vi "Raycaster_DrawBackground.vi"(7 "column":u32) -> ()   [LabVIEW 2020]
uses:
  <vilib>/Platform/TimedLoop/XDataNode/timing_clust.ctl
  <vilib>/Platform/TimedLoop/XDataNode/nitl_modes.ctl
  <vilib>/Platform/TimedLoop/XDataNode/wakeup.ctl
  <vilib>/rvi/Emulation/niFpgaEmulationIsFPGAContextNoSignature.vi
  <vilib>/rvi/DataTransferAndStorage/Container/Common/niFpgaContainerGetUniqueNameForEmu.vi
  <vilib>/rvi/Memory/Memory_Emulation/niFpgaMemoryEmulationCacheClearOnFirstRun.vi
  <vilib>/rvi/Memory/Memory_Emulation/nirvimemoryEmulationManagerCache_MakeExclusive.vi
  <vilib>/rvi/Memory/Memory_Emulation/niFpgaMemoryEmulationValidateCache.vi
  <vilib>/rvi/Memory/Memory_Emulation/nirvimemoryEmulationManagerCache_InsertValue.vi
  <vilib>/Utility/error.llb/Clear Errors.vi
  <vilib>/rvi/Memory/Memory_Emulation/nirvimemoryEmulationManagerCache_ReleaseExclusive.vi
  <vilib>/rvi/Memory/Memory_Emulation/nirvimemoryEmulationManagerCache_GetValue.vi
  <vilib>/rvi/Memory/Memory_Emulation/nirvimemoryEmulationManagerCache_SetValue.vi
  <vilib>/rvi/Emulation/niFpgaProcessEmulError.vi
  <vilib>/rvi/Emulation/niFpgaSctlEmulationGetInTimedLoop.vi
  <vilib>/rvi/Emulation/niFpgaEmulationReportErrorSimple.vi
  <vilib>/rvi/Emulation/niFpgaGetClockAttributes.vi
  <vilib>/rvi/Emulation/niFpgaCriticalErrorInLSC.vi
  <vilib>/rvi/Memory/Memory_Emulation/nirvimemoryEmulation.vi
  <vilib>/rvi/Memory/Memory_Emulation/nirvimemoryFastEmulation.vi
  <vilib>/rvi/errors/nirviReportUnexpectedCaseInternalError (U32).vi
  <vilib>/rvi/DataTransferAndStorage/Container/XNode/niFpgaContainer.xnode
  <vilib>/rvi/DataTransferAndStorage/Register/Emulation/niFpgaRegisterEmulation.vi
  <vilib>/Platform/TimedLoop/XDataNode/XDataNode.xnode
  <vilib>/Platform/TimedLoop/XDataNode/XDNodeRunTimeDep.lvlib
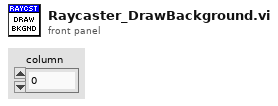
[diagram p1: front panel]
types:
  T1 = typedef "XDNodeRunTimeDep.lvlib/timing_clust.ctl" = cluster{"Expected End [f-1]":u64, "Actual End [f-1]":u64, "Finished Late? [f-1]":bool, "Expected End [i-1]":u64, "Actual End [i-1]":u64, "Finished Late? [i-1]":bool, "Expected Start [i]":u64, "Actual Start [i]":u64, "Expected Start [f]":u64, "Actual Start [f]":u64, "Source Name":string, "Structure Name":string, "Period":i64, "Deadline":i64, "Offset":i64, "Start":i64, "Priority":i32, "Timeout":i32, "Mode":T2, "Wakeup Reason":T3, "Error":errorcluster, "Source Type":string, "Secondary Source Type":string, "Global End Time":u64, "Global Start Time":u64, "Frame Duration":u64, "Iteration Duration":u64, "Assigned CPU":i32, "I/O Scan Engine Mode":u32}
  T2 = typedef "XDNodeRunTimeDep.lvlib/nitl_modes.ctl" = enum32{"No Change", "Process missed periods, maintain original phase", "Discard missed periods, maintain original phase", "Process missed periods, ignore original phase", "Discard missed periods, ignore original phase"}
  T3 = typedef "XDNodeRunTimeDep.lvlib/wakeup.ctl" = enum32{"Normal", "Aborted", "Asynchronous wakeup", "Timing source error", "Timed loop error", "Timeout"}
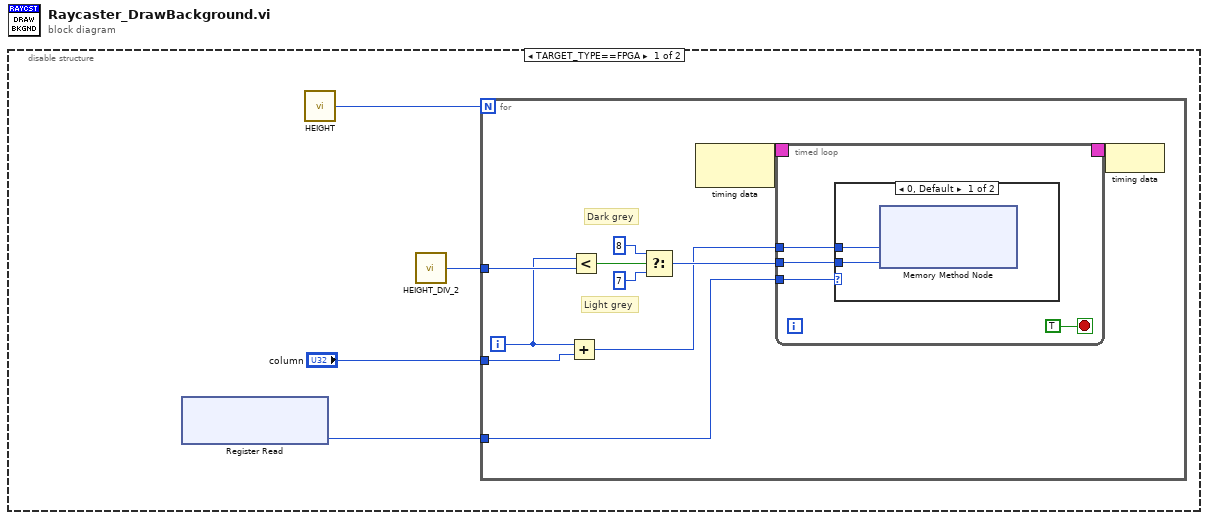
[diagram p0: block diagram]
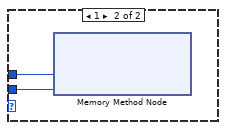
[diagram p2: hidden frame]
diagram:
  n1 = disable-structure shown="TARGET_TYPE==FPGA" {
    frame condition #0 (active) {
      n2 = xnode ("Register Read")() -> ("Data"=w4:u8)  [unwired: 1 in, 1 out]
      n3 = call "HEIGHT.vi"() -> ("HEIGHT"=w2:i16)
      n4 = call "HEIGHT_DIV_2.vi"() -> ("HEIGHT_DIV_2"=w3:i16)
      n5 = for {
        N: w2 -> [_]
        tunnel: w4 -> [w15]
        tunnel: w3 -> [w14]
        tunnel: "column" -> [w6]
        i -> [w7]
        # "Light grey"
        # "Dark grey"
        n6 = Add(x=w7, y=w6) -> (x+y=w5:u32)
        n7 = Less?(x=w7, y=w14) -> (x < y?=w13:bool)
        n8 = Select(t=u8 8, s=w13, f=u8 7) -> (s? t:f=w10:u8)
        n9 = node-c288() -> (w9:T1)  [unwired: 1 in]
        n10 = timed-loop {
          timing: w9 -> [_]
          timing-out: [_] -> w8
          tunnel: w5 -> [w19]
          tunnel: w15 -> [w18]
          tunnel: w10 -> [w17]
          stop <- TRUE stop-if-true
          n11 = case shown="0, Default" w18 {
            tunnel: w19 -> [w21 w23]
            tunnel: w17 -> [w20 w22]
            frame 0, Default {
              n12 = xnode ("Memory Method Node")("Address"=w21, "Data"=w20) -> ()  [unwired: 1 in, 1 out]
            }
            frame 1 {
              n13 = xnode ("Memory Method Node")("Address"=w23, "Data"=w22) -> ()  [unwired: 1 in, 1 out]
            }
          }
        }
        n14 = node-c288(w8) -> ()
      }
    }
    frame condition #1 {
    }
  }
